vi "Teleop.vi"(10 "Match Info":T1={"Autonomous Elapsed Seconds"=0.0, "TeleOp Elapsed Seconds"=0.0, "Disabled Elapsed Seconds"=0.0, "Visited Autonomous"=FALSE, "Visited TeleOp"=FALSE, "Visited Disabled"=FALSE, "Autonomous Settings"={"Autonomous Style"=enum."Independent", "VI Refnum"=refnum}}, 11 "Call Context":T2) -> ()   [LabVIEW 2018]
doc: "This VI is called for each TeleOp packet received from the DS where the robot is not disabled. It is often used to read from the joysticks and update I/O or to update setpoints for timed control loops. It should complete and return within 20 milliseconds or it may miss DS packets."
uses:
  <vilib>/Rock Robotics/WPI/DriverStation/WPI_DriverStationDerivedRobotMode.ctl
  <vilib>/Rock Robotics/WPI/DriverStation/WPI_DriverStationMatch Info.ctl
  <vilib>/Rock Robotics/Network Tables/NT Read Boolean.vi
  <vilib>/Rock Robotics/Network Tables/NT Read Number.vi
  <vilib>/Rock Robotics/WPI/Utilities/WPI_GetSetVariantRefNum.vi
  <vilib>/Rock Robotics/Network Tables/NT Write Boolean Array.vi
  <vilib>/Rock Robotics/Network Tables/NT Write Numeric Array.vi
  <vilib>/Rock Robotics/Network Tables/NT Read Numeric Array.vi
  <vilib>/Rock Robotics/Network Tables/NT Write Boolean.vi
panel:
  in  "Motor Stall":dbl format="%#_13g"
  out "Sample Slider 0":dbl(slide) scale=0.0..5.0
  out "Sample Boolean 1":bool
  out "Sample Boolean 0":bool
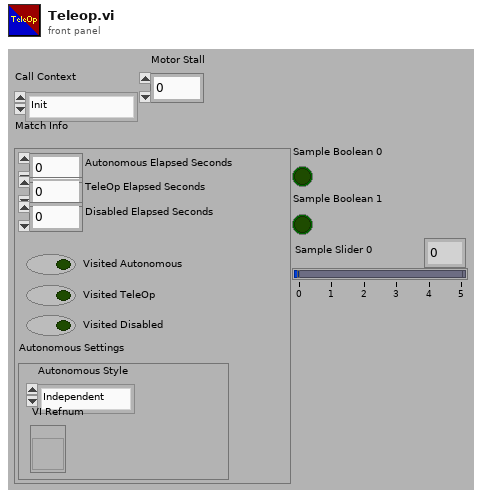
[diagram p1: front panel]
types:
  T1 = typedef "WPI_DriverStationMatch Info.ctl" = cluster{"Autonomous Elapsed Seconds":dbl, "TeleOp Elapsed Seconds":dbl, "Disabled Elapsed Seconds":dbl, "Visited Autonomous":bool, "Visited TeleOp":bool, "Visited Disabled":bool, "Autonomous Settings":cluster{"Autonomous Style":enum16{"Iterative", "Independent"}, "VI Refnum":refnum<vi>}}
  T2 = typedef "WPI_DriverStationDerivedRobotMode.ctl" = enum16{"Init", "Execute", "Stop"}
  T3 = typedef "WPI_JoystickDevRef.ctl" = cluster{"Device":T4}
  T4 = typedef "WPI_JoystickDeviceEnum.ctl" = enum16{"USB 0", "USB 1", "USB 2", "USB 3", "USB 4", "USB 5"}
  T5 = typedef "WPI_MotorControlDeviceRef.ctl" = cluster{"DeviceStatus":errorcluster, "Type":T6, "PWM":cluster{"PWM Channel":T7, "DeadBand":T8}, "CAN":cluster{"Device Number":u8, "SetOutput VI Ref":variant, "GetOutput VI Ref":variant, "Enable VI Ref":variant, "Disable VI Ref":variant, "Data":variant}, "Invert":bool, "DIO PWM":cluster{"PWM \"Enable\" Channel":T7, "DIOChannel":T9, "PWM Rate":dbl}}
  T6 = typedef "WPI_MotorControlType.ctl" = enum16{"PWM", "CAN", "DIO PWM"}
  T7 = typedef "FPGA_DIOPWMChannel.ctl" = enum8{"PWM 0", "PWM 1", "PWM 2", "PWM 3", "PWM 4", "PWM 5", "PWM 6", "PWM 7", "PWM 8", "PWM 9", "PWM MXP 0", "PWM MXP 1", "PWM MXP 2", "PWM MXP 3", "PWM MXP 4", "PWM MXP 5", "PWM MXP 6", "PWM MXP 7", "PWM MXP 8", "PWM MXP 9", "Invalid"}
  T8 = typedef "WPI_PWMDeadband.ctl" = cluster{"Name":string, "maxPositivePwm":i32, "minPositivePwm":i32, "centerPwm":i32, "maxNegativePwm":i32, "minNegativePwm":i32, "angularRange":u16}
  T9 = typedef "FPGA_DIOChannel.ctl" = enum8{"DIO 0", "DIO 1", "DIO 2", "DIO 3", "DIO 4", "DIO 5", "DIO 6", "DIO 7", "DIO 8", "DIO 9", "DIO MXP 0", "DIO MXP 1", "DIO MXP 2", "DIO MXP 3", "DIO MXP 4", "DIO MXP 5", "DIO MXP 6", "DIO MXP 7", "DIO MXP 8", "DIO MXP 9", "DIO MXP 10", "DIO MXP 11", "DIO MXP 12", "DIO MXP 13", "DIO MXP 14", "DIO MXP 15", "SPI Port CS1", "SPI Port CS2", "SPI Port CS3", "SPI Port MISO", "SPI Port MOSI", "Invalid"}
  T10 = typedef "WPI_RobotDriveDevRef.ctl" = cluster{"DevStatus":errorcluster, "Motors[]":T5[], "Square Inputs":bool, "Max Output":dbl}
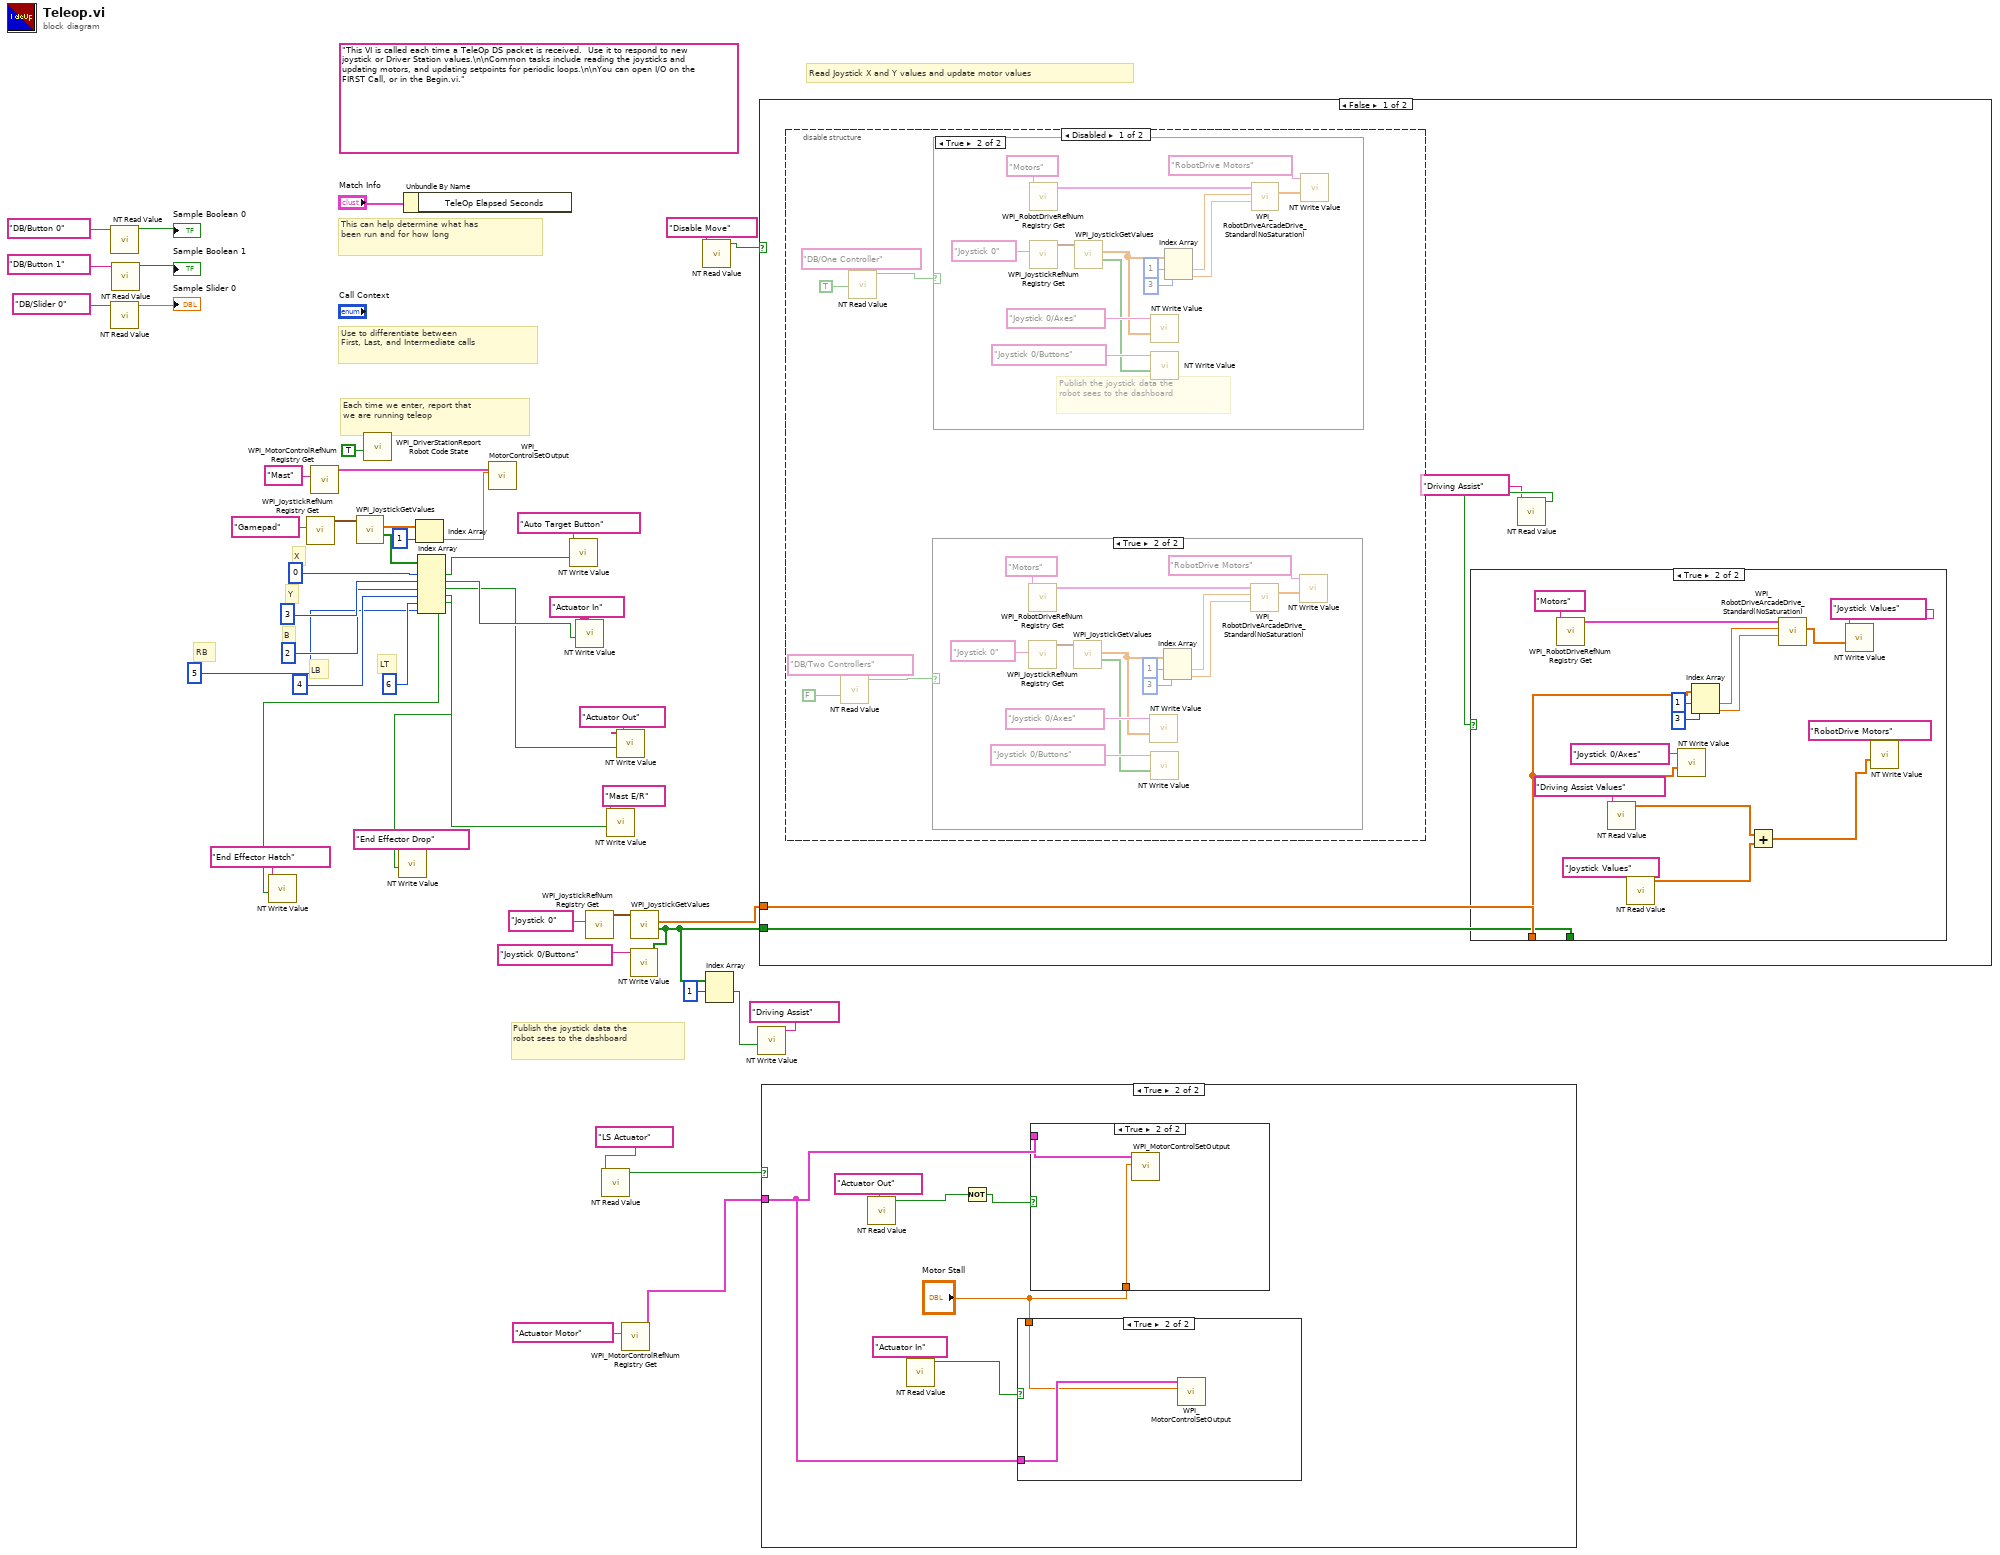
[diagram p0: block diagram]
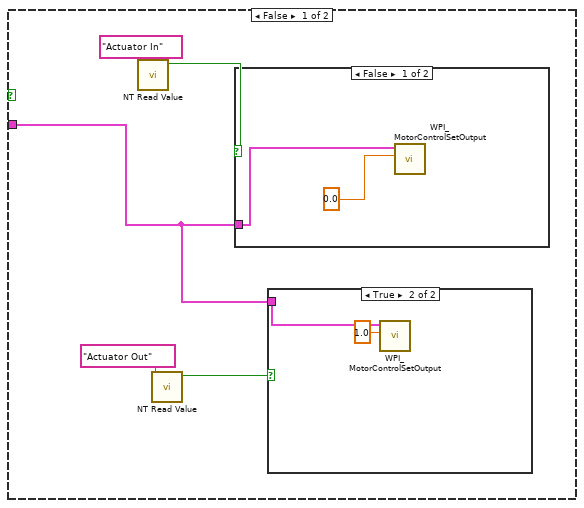
[diagram p2: hidden frame]
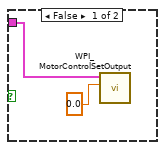
[diagram p3: hidden frame]
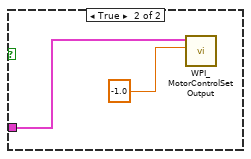
[diagram p4: hidden frame]
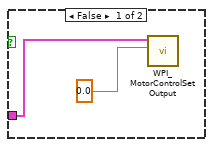
[diagram p5: hidden frame]
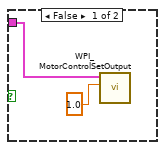
[diagram p6: hidden frame]
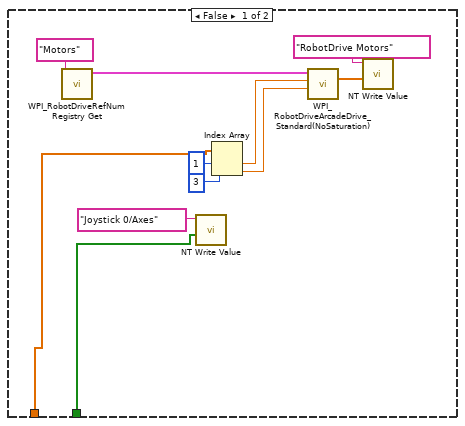
[diagram p7: hidden frame]
diagram:
  (unwired) "This VI is called each time a TeleOp DS packet is received.  Use it to respond to new joystick or Driver Station values.\n\nCommon tasks include reading the joysticks and updating motors, and updating setpoints for periodic loops.\n\nYou can open I/O on the FIRST Call, or in the Begin.vi."
  # "RB"
  # "LT"
  # "LB"
  # "Publish the joystick data the\nrobot sees to the dashboard"
  # "B"
  # "X"
  # "Y"
  # "Each time we enter, report that\nwe are running teleop"
  # "Use to differentiate between\nFirst, Last, and Intermediate calls"
  # "This can help determine what has\nbeen run and for how long"
  # "Read Joystick X and Y values and update motor values"
  n1 = call-poly <vilib>:"NT Read Value.vi"("Name"="DB/Button 0" ("refnum name")) -> ("Boolean"=→"Sample Boolean 0":bool)  [unwired: 9 in, 1 out]
  n2 = call-poly <vilib>:"NT Read Value.vi"("Name"="DB/Slider 0" ("refnum name")) -> ("Numeric"=→"Sample Slider 0":dbl)  [unwired: 9 in, 1 out]
  n3 = call-poly <vilib>:"NT Read Value.vi"("Name"="DB/Button 1" ("refnum name")) -> ("Boolean"=→"Sample Boolean 1":bool)  [unwired: 9 in, 1 out]
  n4 = call <vilib>:"WPI_JoystickRefNum Registry Get.vi"("refnum name"="Gamepad") -> ("JoystickDevRef"=w37:T3)  [unwired: 9 in, 1 out]
  n5 = call <vilib>:"WPI_MotorControlRefNum Registry Get.vi"("refnum name"="Mast") -> ("MotorControlDevRef"=w39:T5)  [unwired: 9 in, 1 out]
  n6 = call <vilib>:"WPI_JoystickGetValues.vi"("JoystickDevRef"=w37) -> ("Buttons"=w31:bool[], "Axes"=w36:dbl[])  [unwired: 6 in, 3 out]
  n7 = call <vilib>:"WPI_DriverStationReport Robot Code State.vi"("TeleOp"=TRUE ("Autonomous")) -> ()  [unwired: 10 in, 1 out]
  n8 = Unbundle By Name("Match Info") -> ()  [unwired: 1 out]
  n9 = Index Array(array=w36, index=1) -> (element=w35:dbl)
  n10 = Index Array(array=w31, index #1=0 ("index"), index #2=3 ("index"), index #3=2 ("index"), index #4=4 ("index"), index #5=6 ("index"), index #6=5 ("index")) -> (element #1=w29:bool, element #2=w23:bool, element #3=w20:bool, element #4=w9:bool, element #5=w7:bool, element #6=w5:bool)
  n11 = call-poly <vilib>:"NT Write Value.vi"("Boolean"=w5, "Name"="End Effector Hatch") -> ()  [unwired: 9 in, 1 out]
  n12 = call-poly <vilib>:"NT Write Value.vi"("Boolean"=w7, "Name"="End Effector Drop") -> ()  [unwired: 9 in, 1 out]
  n13 = call <vilib>:"WPI_MotorControlSetOutput.vi"("Output"=w35, "MotorControlDevRef"=w39) -> ()  [unwired: 7 in, 3 out]
  n14 = call-poly <vilib>:"NT Write Value.vi"("Boolean"=w29, "Name"="Auto Target Button") -> ()  [unwired: 9 in, 1 out]
  n15 = call-poly <vilib>:"NT Write Value.vi"("Boolean"=w23, "Name"="Actuator In") -> ()  [unwired: 9 in, 1 out]
  n16 = call <vilib>:"WPI_JoystickRefNum Registry Get.vi"("refnum name"="Joystick 0") -> ("JoystickDevRef"=w17:T3)  [unwired: 1 in, 9 out]
  n17 = call-poly <vilib>:"NT Read Value.vi"("Name"="LS Actuator") -> ("Boolean"=w26:bool)  [unwired: 9 in, 1 out]
  n18 = call-poly <vilib>:"NT Write Value.vi"("Boolean"=w9, "Name"="Mast E/R") -> ()  [unwired: 9 in, 1 out]
  n19 = call-poly <vilib>:"NT Write Value.vi"("Boolean"=w20, "Name"="Actuator Out") -> ()  [unwired: 9 in, 1 out]
  n20 = call <vilib>:"WPI_MotorControlRefNum Registry Get.vi"("refnum name"="Actuator Motor") -> ("MotorControlDevRef"=w18:T5)  [unwired: 9 in, 1 out]
  n21 = call <vilib>:"WPI_JoystickGetValues.vi"("JoystickDevRef"=w17) -> ("Buttons"=w13:bool[], "Axes"=w15:dbl[])  [unwired: 6 in, 3 out]
  n22 = call-poly <vilib>:"NT Write Value.vi"("Boolean Array"=w13, "Name"="Joystick 0/Buttons") -> ()  [unwired: 9 in, 1 out]
  n23 = call-poly <vilib>:"NT Read Value.vi"("Name"="Disable Move") -> ("Boolean"=w33:bool)  [unwired: 9 in, 1 out]
  n24 = Index Array(array=w13, index #1=1 ("index")) -> (element #1=w11:bool)  [unwired: 1 in, 1 out]
  n25 = call-poly <vilib>:"NT Write Value.vi"("Boolean"=w11, "Name"="Driving Assist") -> ()  [unwired: 9 in, 1 out]
  n26 = case shown="False" w33 {
    tunnel: w13 -> [w51 _]
    tunnel: w15 -> [w52 _]
    frame False {
      n27 = disable-structure shown="Disabled" {
        frame Disabled {
          n28 = call-poly <vilib>:"NT Read Value.vi"("Default Value"=FALSE, "Name"="DB/Two Controllers") -> ("Boolean"=w83:bool)  [unwired: 8 in, 1 out]
          n29 = call-poly <vilib>:"NT Read Value.vi"("Default Value"=TRUE, "Name"="DB/One Controller") -> ("Boolean"=w85:bool)  [unwired: 8 in, 1 out]
          n30 = case shown="True" w83 {
            frame False {
            }
            frame True {
              n31 = call <vilib>:"WPI_RobotDriveRefNum Registry Get.vi"("refnum name"="Motors") -> ("RobotDriveDevRef"=w98:T10)  [unwired: 1 in, 9 out]
              n32 = call <vilib>:"WPI_JoystickRefNum Registry Get.vi"("refnum name"="Joystick 0") -> ("JoystickDevRef"=w96:T3)  [unwired: 1 in, 9 out]
              n33 = call <vilib>:"WPI_JoystickGetValues.vi"("JoystickDevRef"=w96) -> ("Buttons"=w91:bool[], "Axes"=w92:dbl[])  [unwired: 6 in, 3 out]
              n34 = call-poly <vilib>:"NT Write Value.vi"("Numeric Array"=w92, "Name"="Joystick 0/Axes") -> ()  [unwired: 9 in, 1 out]
              n35 = call-poly <vilib>:"NT Write Value.vi"("Boolean Array"=w91, "Name"="Joystick 0/Buttons") -> ()  [unwired: 9 in, 1 out]
              n36 = Index Array(array=w92, index #1=1 ("index"), index #2=3 ("index")) -> (element #1=w97:dbl, element #2=w95:dbl)
              n37 = call <vilib>:"WPI_RobotDriveArcadeDrive_Standard(NoSaturation).vi"("Y axis value"=w95, "X axis value"=w97, "RobotDriveDevRef"=w98) -> ("Motor Values"=w90:dbl[])  [unwired: 1 in, 7 out]
              n38 = call-poly <vilib>:"NT Write Value.vi"("Numeric Array"=w90, "Name"="RobotDrive Motors") -> ()  [unwired: 9 in, 1 out]
            }
          }
          n39 = case shown="True" w85 {
            frame False {
            }
            frame True {
              # "Publish the joystick data the\nrobot sees to the dashboard"
              n40 = call <vilib>:"WPI_RobotDriveRefNum Registry Get.vi"("refnum name"="Motors") -> ("RobotDriveDevRef"=w112:T10)  [unwired: 1 in, 9 out]
              n41 = call <vilib>:"WPI_JoystickRefNum Registry Get.vi"("refnum name"="Joystick 0") -> ("JoystickDevRef"=w110:T3)  [unwired: 1 in, 9 out]
              n42 = call <vilib>:"WPI_JoystickGetValues.vi"("JoystickDevRef"=w110) -> ("Buttons"=w105:bool[], "Axes"=w106:dbl[])  [unwired: 6 in, 3 out]
              n43 = call-poly <vilib>:"NT Write Value.vi"("Numeric Array"=w106, "Name"="Joystick 0/Axes") -> ()  [unwired: 9 in, 1 out]
              n44 = call-poly <vilib>:"NT Write Value.vi"("Boolean Array"=w105, "Name"="Joystick 0/Buttons") -> ()  [unwired: 9 in, 1 out]
              n45 = Index Array(array=w106, index #1=1 ("index"), index #2=3 ("index")) -> (element #1=w111:dbl, element #2=w109:dbl)
              n46 = call <vilib>:"WPI_RobotDriveArcadeDrive_Standard(NoSaturation).vi"("Y axis value"=w109, "X axis value"=w111, "RobotDriveDevRef"=w112) -> ("Motor Values"=w104:dbl[])  [unwired: 1 in, 7 out]
              n47 = call-poly <vilib>:"NT Write Value.vi"("Numeric Array"=w104, "Name"="RobotDrive Motors") -> ()  [unwired: 9 in, 1 out]
            }
          }
        }
        frame Enabled {
        }
      }
      n48 = call-poly <vilib>:"NT Read Value.vi"("Name"="Driving Assist") -> ("Boolean"=w50:bool)  [unwired: 9 in, 1 out]
      n49 = case shown="True" w50 {
        tunnel: w52 -> [w54 w72]
        tunnel: w51 -> [w53 _]
        frame False {
          n50 = call <vilib>:"WPI_RobotDriveRefNum Registry Get.vi"("refnum name"="Motors") -> ("RobotDriveDevRef"=w62:T10)  [unwired: 1 in, 9 out]
          n51 = call-poly <vilib>:"NT Write Value.vi"("Boolean Array"=w53, "Name"="Joystick 0/Axes") -> ()  [unwired: 9 in, 1 out]
          n52 = Index Array(array=w54, index #1=1 ("index"), index #2=3 ("index")) -> (element #1=w61:dbl, element #2=w60:dbl)
          n53 = call <vilib>:"WPI_RobotDriveArcadeDrive_Standard(NoSaturation).vi"("Y axis value"=w60, "X axis value"=w61, "RobotDriveDevRef"=w62) -> ("Motor Values"=w58:dbl[])  [unwired: 1 in, 7 out]
          n54 = call-poly <vilib>:"NT Write Value.vi"("Numeric Array"=w58, "Name"="RobotDrive Motors") -> ()  [unwired: 9 in, 1 out]
        }
        frame True {
          n55 = call <vilib>:"WPI_RobotDriveRefNum Registry Get.vi"("refnum name"="Motors") -> ("RobotDriveDevRef"=w78:T10)  [unwired: 1 in, 9 out]
          n56 = call-poly <vilib>:"NT Read Value.vi"("Name"="Driving Assist Values") -> ("Numeric Array"=w67:dbl[])  [unwired: 9 in, 1 out]
          n57 = call-poly <vilib>:"NT Read Value.vi"("Name"="Joystick Values") -> ("Numeric Array"=w66:dbl[])  [unwired: 9 in, 1 out]
          n58 = call-poly <vilib>:"NT Write Value.vi"("Numeric Array"=w72, "Name"="Joystick 0/Axes") -> ()  [unwired: 9 in, 1 out]
          n59 = Index Array(array=w72, index #1=1 ("index"), index #2=3 ("index")) -> (element #1=w77:dbl, element #2=w76:dbl)
          n60 = Add(x=w67, y=w66) -> (x+y=w64:dbl[])
          n61 = call <vilib>:"WPI_RobotDriveArcadeDrive_Standard(NoSaturation).vi"("Y axis value"=w76, "X axis value"=w77, "RobotDriveDevRef"=w78) -> ("Motor Values"=w70:dbl[])  [unwired: 1 in, 7 out]
          n62 = call-poly <vilib>:"NT Write Value.vi"("Numeric Array"=w70, "Name"="Joystick Values") -> ()  [unwired: 9 in, 1 out]
          n63 = call-poly <vilib>:"NT Write Value.vi"("Numeric Array"=w64, "Name"="RobotDrive Motors") -> ()  [unwired: 9 in, 1 out]
        }
      }
    }
    frame True {
    }
  }
  n64 = case shown="True" w26 {
    tunnel: w18 -> [w114 w128]
    frame False {
      n65 = call-poly <vilib>:"NT Read Value.vi"("Name"="Actuator In") -> ("Boolean"=w117:bool)  [unwired: 9 in, 1 out]
      n66 = call-poly <vilib>:"NT Read Value.vi"("Name"="Actuator Out") -> ("Boolean"=w116:bool)  [unwired: 9 in, 1 out]
      n67 = case shown="False" w117 {
        tunnel: w114 -> [w123 w125]
        frame False {
          n68 = call <vilib>:"WPI_MotorControlSetOutput.vi"("Output"=0.0, "MotorControlDevRef"=w123) -> ()  [unwired: 7 in, 3 out]
        }
        frame True {
          n69 = call <vilib>:"WPI_MotorControlSetOutput.vi"("Output"=-1.0, "MotorControlDevRef"=w125) -> ()  [unwired: 7 in, 3 out]
        }
      }
      n70 = case shown="True" w116 {
        tunnel: w114 -> [w120 w122]
        frame False {
          n71 = call <vilib>:"WPI_MotorControlSetOutput.vi"("Output"=0.0, "MotorControlDevRef"=w120) -> ()  [unwired: 7 in, 3 out]
        }
        frame True {
          n72 = call <vilib>:"WPI_MotorControlSetOutput.vi"("Output"=1.0, "MotorControlDevRef"=w122) -> ()  [unwired: 7 in, 3 out]
        }
      }
    }
    frame True {
      n73 = call-poly <vilib>:"NT Read Value.vi"("Name"="Actuator Out") -> ("Boolean"=w132:bool)  [unwired: 9 in, 1 out]
      n74 = call-poly <vilib>:"NT Read Value.vi"("Name"="Actuator In") -> ("Boolean"=w129:bool)  [unwired: 9 in, 1 out]
      n75 = Not(x=w132) -> (.not. x?=w131:bool)
      n76 = case shown="True" w129 {
        tunnel: w128 -> [w134 w137]
        tunnel: "Motor Stall" -> [_ w136]
        frame False {
          n77 = call <vilib>:"WPI_MotorControlSetOutput.vi"("Output"=0.0, "MotorControlDevRef"=w134) -> ()  [unwired: 7 in, 3 out]
        }
        frame True {
          n78 = call <vilib>:"WPI_MotorControlSetOutput.vi"("Output"=w136, "MotorControlDevRef"=w137) -> ()  [unwired: 7 in, 3 out]
        }
      }
      n79 = case shown="True" w131 {
        tunnel: w128 -> [w139 w141]
        tunnel: "Motor Stall" -> [_ w140]
        frame False {
          n80 = call <vilib>:"WPI_MotorControlSetOutput.vi"("Output"=1.0, "MotorControlDevRef"=w139) -> ()  [unwired: 7 in, 3 out]
        }
        frame True {
          n81 = call <vilib>:"WPI_MotorControlSetOutput.vi"("Output"=w140, "MotorControlDevRef"=w141) -> ()  [unwired: 7 in, 3 out]
        }
      }
    }
  }
